vi "Config.vi"(0 "SharedVariableWrapper in":refnum<class "SharedVariableWrapper.lvclass">, 5 "host":string="localhost", 7 "lib":string="TrendAnaliserEng", 9 "update timeout":dbl, 11 "error in":errorcluster) -> (4 "SharedVariableWrapper":refnum<class "SharedVariableWrapper.lvclass">, 15 "error out":errorcluster)   [LabVIEW 2019, in "SharedVariableWrapper.lvclass"]
uses:
  SharedVariableWrapper.lvclass
  SharedVariableWrapper.lvclass/SharedVariableWrapper.ctl
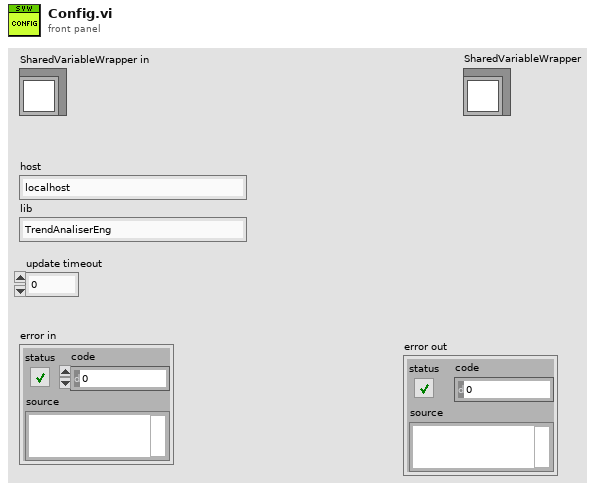
[diagram p1: front panel]
types:
  T1 = typedef "SharedVariableWrapper.lvclass/Config.ctl" = cluster{"connection str":string, "timeout":dbl, "ip":string}
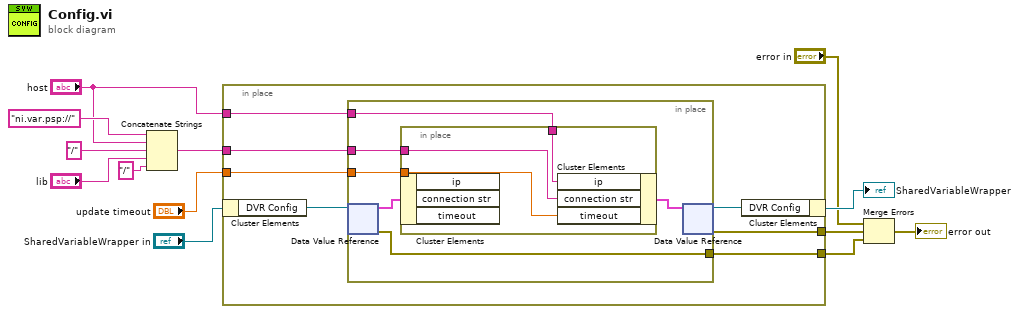
[diagram p0: block diagram]
diagram:
  n1 = Concatenate Strings("ni.var.psp://" ("string"), "host", "/" ("string"), "lib", "/" ("string")) -> (w8:string)
  n2 = in-place {
    in-place-border: w8 -> [w19]
    in-place-border: [w17] -> w6
    in-place-border: [w16] -> w5
    in-place-border: "update timeout" -> [w15]
    in-place-border: "host" -> [w14]
    n3 = in-place-cluster #1("SharedVariableWrapper in") -> ("DVR Config"=w20:refnum<data-value>)
    n4 = in-place {
      in-place-border: w19 -> [w23]
      in-place-border: [w26] -> w16
      in-place-border: w15 -> [w22]
      in-place-border: w14 -> [w21]
      n5 = in-place-dvr #2(w20) -> (w25:T1, w26:errorcluster)
      n6 = in-place {
        in-place-border: w23 -> [w29]
        in-place-border: w22 -> [w28]
        in-place-border: w21 -> [w27]
        n7 = in-place-cluster #3(w25) -> ()  [unwired: 3 out]
        n8 = in-place-cluster #3("ip"=w27, "connection str"=w29, "timeout"=w28) -> (w24:T1)
      }
      n9 = in-place-dvr #2(w24) -> (w18:refnum<data-value>, w17:errorcluster)
    }
    n10 = in-place-cluster #1("DVR Config"=w18) -> (→"SharedVariableWrapper":refnum<class "SharedVariableWrapper.lvclass">)
  }
  n11 = Merge Errors("error in", w6, w5) -> (→"error out":errorcluster)
